vi "Execute Generic Command.vi"(0 "session in":refnum<k21>, 5 "resources":string, 7 "command":refnum<k21>, 11 "error in (no error)":errorcluster, 12 "timeout (10 sec)":dbl=10.0) -> (4 "session out":refnum<k21>, 15 "error out":errorcluster)   [LabVIEW 2020, in "SLSC.lvlib"]
doc: "Executes the specified command on one or multiple devices or physical channels."
uses:
  <vilib>/SLSC/SLSC.lvlib
  nislsclvapi.dll
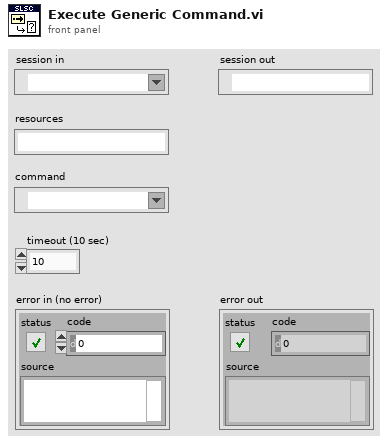
[diagram p1: front panel]
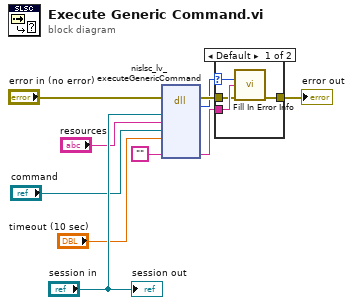
[diagram p0: block diagram]
diagram:
  n1 = dll-call lib="nislsclvapi.*" fn="nislsc_lv_executeGenericCommand"(error in="error in (no error)", "session"="session in", "resources"="resources", "command"="command", "timeout"="timeout (10 sec)", "extendedErrorInfo"="") -> (error out=w6:errorcluster, "return type"=w5:i32, "extendedErrorInfo"=w7:string)  [unwired: 8 in, 1 out]
  n2 = case shown="Default" w5 {
    selector: w5 -> [w14 _]
    tunnel: w7 -> [w13 _]
    tunnel: w6 -> [w12 w15]
    tunnel: [w11 w15] -> w4
    frame Default {
      n3 = call <vilib>:"Fill In Error Info.vi"("status code"=w14, "extended error info"=w13, "error in"=w12) -> ("error out"=w11:errorcluster)  [unwired: 12 in]
    }
    frame 0 {
    }
  }
  "error out" <- w4
  "session out" <- "session in"
